vi "LoadActions.vi"(6 "Array 2":string[](array[string]), 7 "Array":string[](array[string]), 8 "error in (no error)":errorcluster, 9 "Array 4":refnum<vi>[](array[refnum]), 10 "Array 3":refnum<vi>[](array[refnum]), 11 "Item Ref in":T1 format="%.0x") -> (0 "error out":errorcluster, 3 "Item Ref out":T1 format="%.0x")   [LabVIEW 2024, in "Embedded TDMS Logger System Explorer.lvlib"]
uses:
  Embedded TDMS Logger System Explorer.lvlib
  <vilib>/NI VeriStand/Custom Device API/Custom Device Item Ref.ctl
  <vilib>/NI VeriStand/Custom Device API/Get Item Property (Boolean).vi
  <vilib>/NI VeriStand/Custom Device API/Set Item Property (String).vi
  <vilib>/NI VeriStand/Custom Device API/Get Item Property (String).vi
  <vilib>/NI VeriStand/Custom Device API/Custom Device API.lvlib
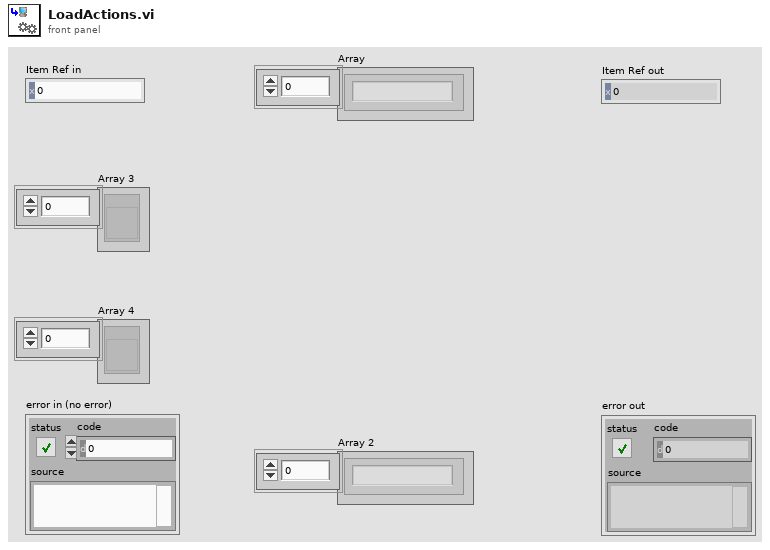
[diagram p1: front panel]
types:
  T1 = typedef "Custom Device API.lvlib/Custom Device Item Ref.ctl" = u64
  T2 = enum8{"Enabled", "Disabled", "Disabled and Grayed Out"}
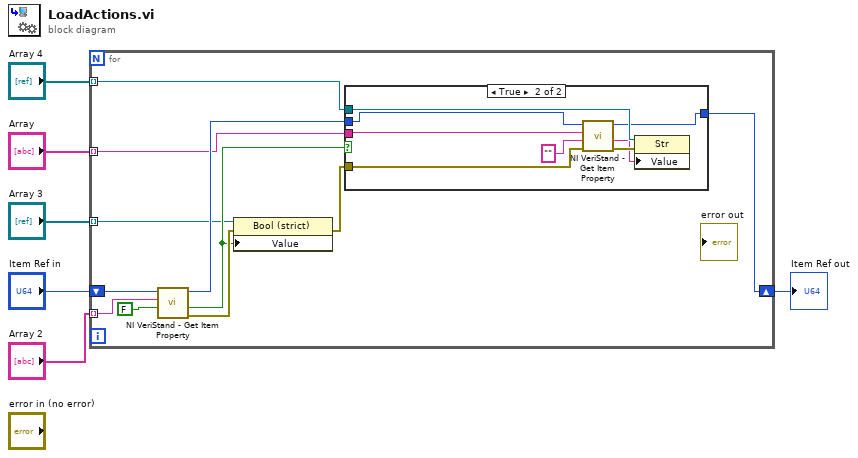
[diagram p0: block diagram]
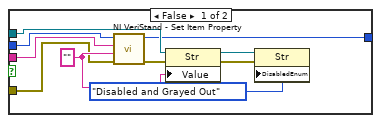
[diagram p2: hidden frame]
diagram:
  n1 = for {
    tunnel: "Array 4" -> [w12] mode=indexing
    tunnel: "Array 3" -> [w11] mode=indexing
    tunnel: "Array 2" -> [w10] mode=indexing
    tunnel: "Array" -> [w8] mode=indexing
    shift-right: [w7] -> w1
    shift-left: "Item Ref in" -> [w9]
    n2 = call-poly <vilib>:"NI VeriStand - Get Item Property.vi"("Default Value"=FALSE, "Property Name"=w10, "Item Ref in"=w9) -> ("error out"=w15:errorcluster, "Value"=w14:bool, "Item Ref out"=w16:T1)  [unwired: 5 in, 1 out]
    n3 = property class="Bool (strict)"(reference=w11, error in=w15, "Value"=w14) -> (error out=w13:errorcluster)  [unwired: 1 out]
    n4 = case shown="True" w14 {
      tunnel: w16 -> [w26 w35]
      tunnel: w13 -> [w24 w34]
      tunnel: w12 -> [w27 w31]
      tunnel: w8 -> [w22 w28]
      tunnel: [w21 w29] -> w7
      frame False {
        w25 = "" ("Default Value")
        n5 = call-poly <vilib>:"NI VeriStand - Set Item Property.vi"("error in (no error)"=w24, "Value"=w25, "Property Name"=w22, "Item Ref in"=w26) -> ("error out"=w23:errorcluster, "Item Ref out"=w21:T1)  [unwired: 5 in, 1 out]
        n6 = property class="Str"(reference=w27, error in=w23, "Value"=w25) -> (reference out=w18:refnum<vi>, error out=w19:errorcluster)
        n7 = property class="Str"(reference=w18, error in=w19, "DisabledEnum"=T2."Disabled and Grayed Out" ("Disabled")) -> ()  [unwired: 2 out]
      }
      frame True {
        n8 = call-poly <vilib>:"NI VeriStand - Get Item Property.vi"("error in (no error)"=w34, "Default Value"="", "Property Name"=w28, "Item Ref in"=w35) -> ("error out"=w32:errorcluster, "Value"=w30:string, "Item Ref out"=w29:T1)  [unwired: 4 in, 1 out]
        n9 = property class="Str"(reference=w31, error in=w32, "Value"=w30) -> ()  [unwired: 2 out]
      }
    }
  }
  "Item Ref out" <- w1
